vi "main_v1.2.vi"() -> ()   [LabVIEW 2012]
uses:
  SensorSettingCtl.ctl
  SensorTypes.ctl
  states.ctl
  globalVariables.vi
  <vilib>/Analysis/NI_AALPro.lvlib
panel:
  out "Array":dbl[](array[numeric])
  in  "end edge / A":dbl=0.5
  in  "start edge / A":dbl=-0.5
  in  "auto slope detect":bool
  out "mean current difference\nto reference / A":dbl[](array[numeric])
  out "charge difference \nto reference / As":dbl[](array[numeric])
  out "lengths of raw times":i32[](array[numeric])
  out "data analysis running":bool
  out "total charge / As":dbl[](array[numeric]) format="%#.2f"
  out "mean current / A":dbl[](array[numeric]) format="%#_5g"
  out "dt":dbl[][](array[numeric])
  out "end-time / s":dbl[](array[numeric]) format="%.3f"
  out "start-time / s":dbl[](array[numeric]) format="%.3f"
  out "calculated sampling rate / s":dbl[](array[numeric]) format="%^#_5e"
  out "zoomed currents":dbl[][](array[numeric])
  out "zoomed times":dbl[][](array[numeric])
  in  "autostart":bool=TRUE
  out "raw currents":dbl[][](array[numeric])
  in  "start-index":i32[](array[numeric]) min=0 step=1
  in  "end-index":i32[](array[numeric])
  out "raw times":dbl[][](array[numeric])
  in  "exit program":bool
  out "meas. time / s":dbl format="%#.1f"
  in  "max. meas. time / s":dbl=8000.0
  out "measuring":bool
  out "currents raw":cluster{dbl[], dbl[]}[](graph)
  out "currents zoomed":cluster{dbl[], dbl[]}[](graph)
  in  "size of result buffer":i32=400000
  in  "Sensor types":T1[](array[typedef])=[enum."IT 600-S (Analogue)", enum."CAB 300-C SP3 (CAN)", enum."difference"]
  in  "Sensor-enabling":T2[](array[typedef])=[{"VISA resource name"="USB0::0x0957::0x2007::MY49004365::INSTR", "use sensor"=TRUE}, {"VISA resource name"="", "use sensor"=TRUE}]
  in  "stop measurement":bool
  in  "start Button":bool
  out "Error Flag":bool
  # "Measurement of Current Sensors from LEM"
  # "Preparation"
  # "reference"
  # "sensor 1"
  # "sensor 2"
  # "Measurement"
  # "Data analysis"
  # "reference"
  # "sensor 1"
  # "sensor 2"
  # "sensor 3"
  # "sensor 4"
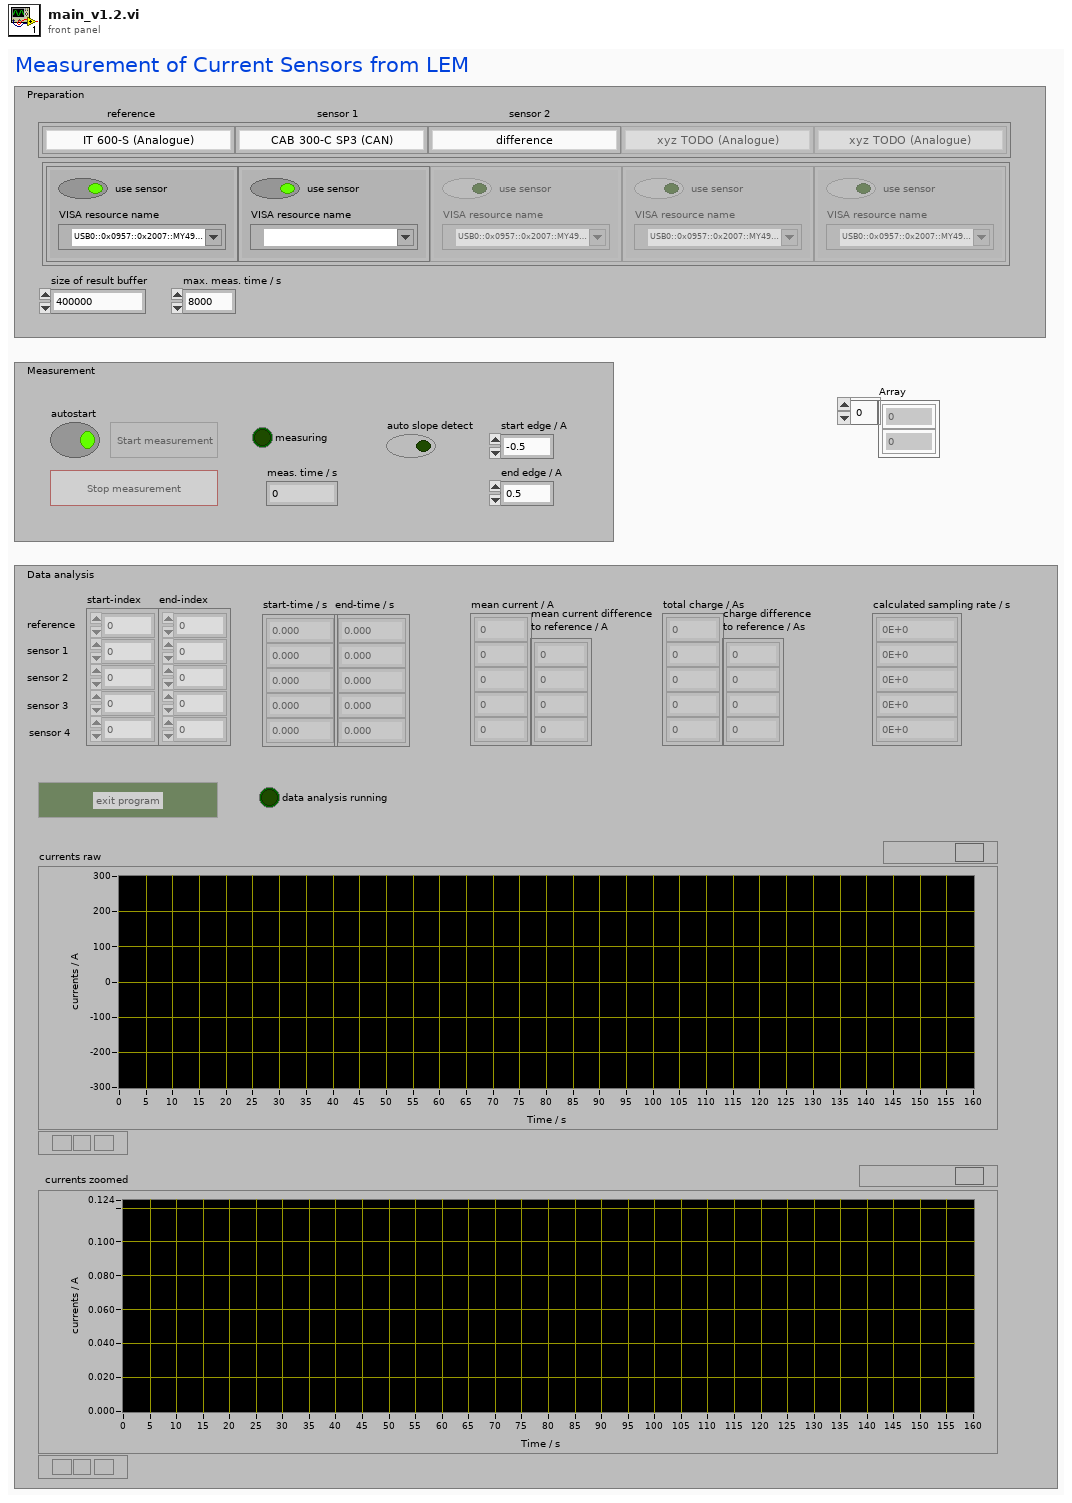
[diagram p1: front panel]
types:
  T1 = typedef "SensorTypes.ctl" = enum16{"IT 600-S (Analogue)", "CAB 300-C SP3 (CAN)", "xyz TODO (PWM)", "xyz TODO (LIN)", "xyz TODO (Analogue)", "difference"}
  T2 = typedef "SensorSettingCtl.ctl" = cluster{"VISA resource name":refnum<visa-resource-name>, "use sensor":bool}
  T3 = typedef "states.ctl" = enum16{"init", "wait for user confirm", "start sensors", "measure", "wait for sensors to finish", "data preparation", "data analysis", "terminate"}
  T4 = enum8{"Enabled", "Disabled", "Disabled and Grayed Out"}
  T5 = typedef "Semaphore RefNum" = refnum<k1>
  T6 = typedef "TimeValue.ctl" = cluster{"Time of measurement":timestamp, "Current value":dbl}
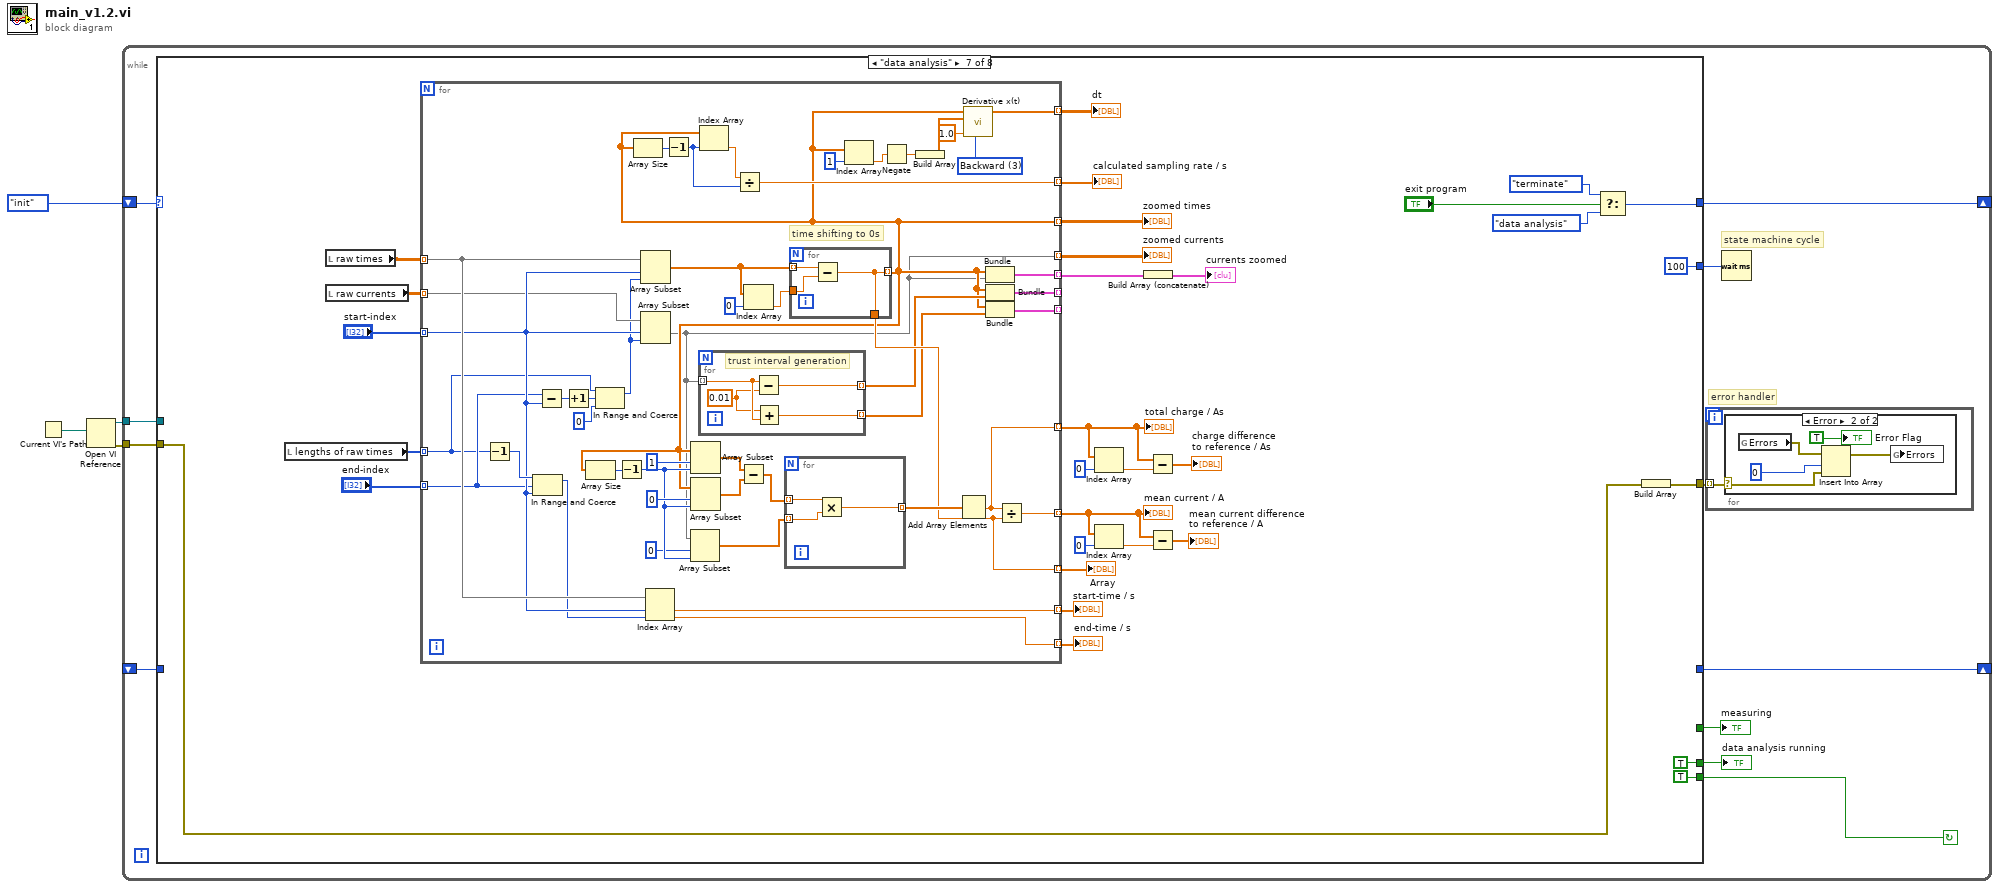
[diagram p0: block diagram]
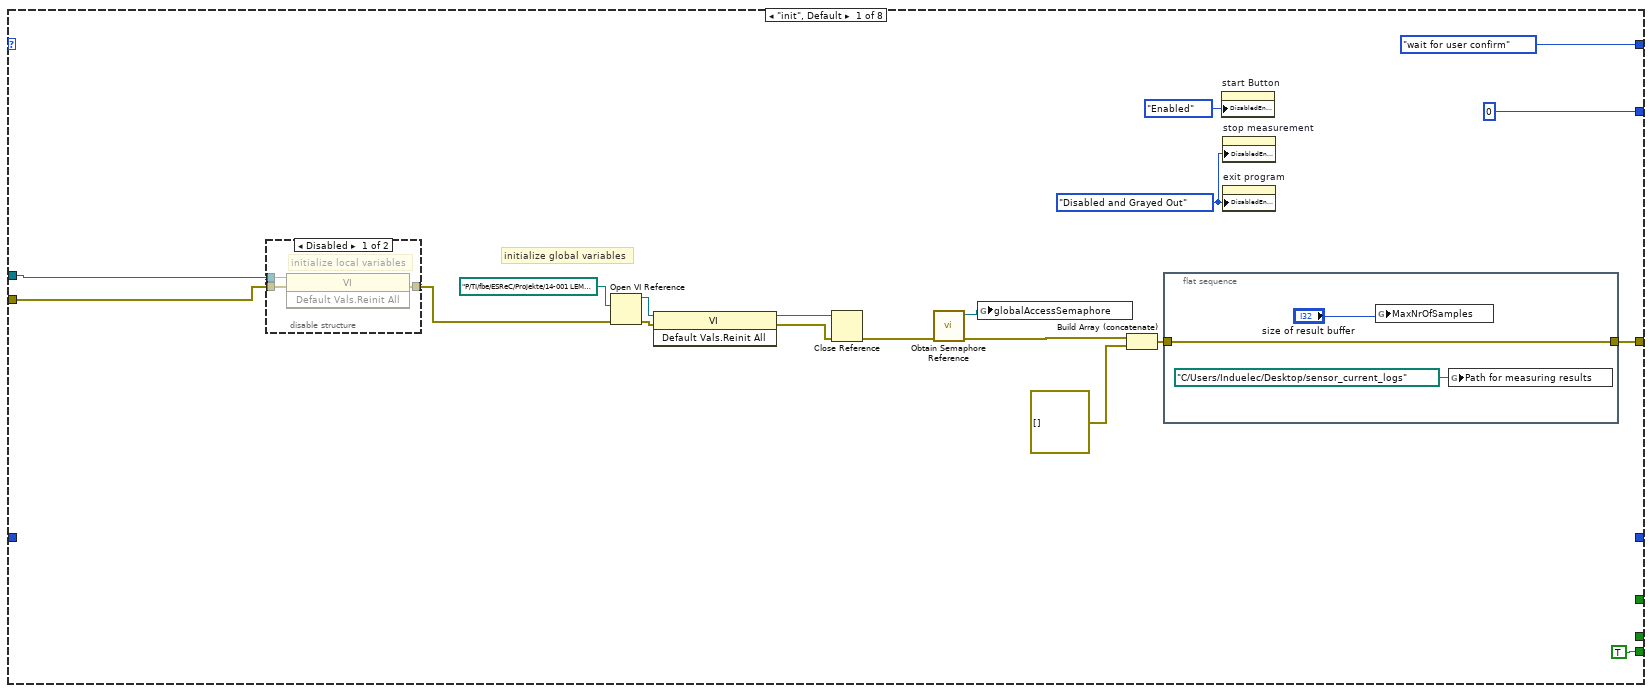
[diagram p3: hidden frame]
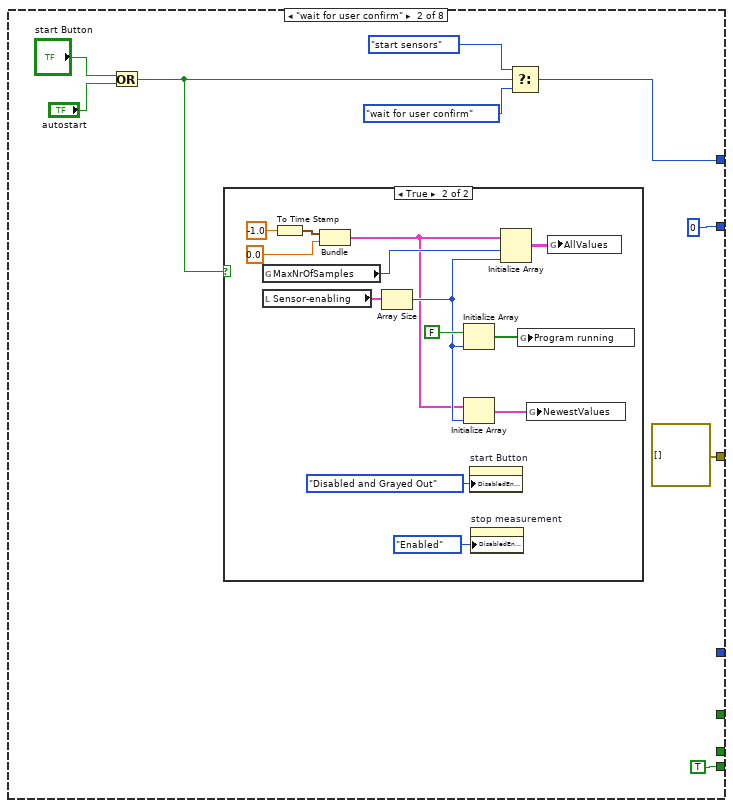
[diagram p5: hidden frame]
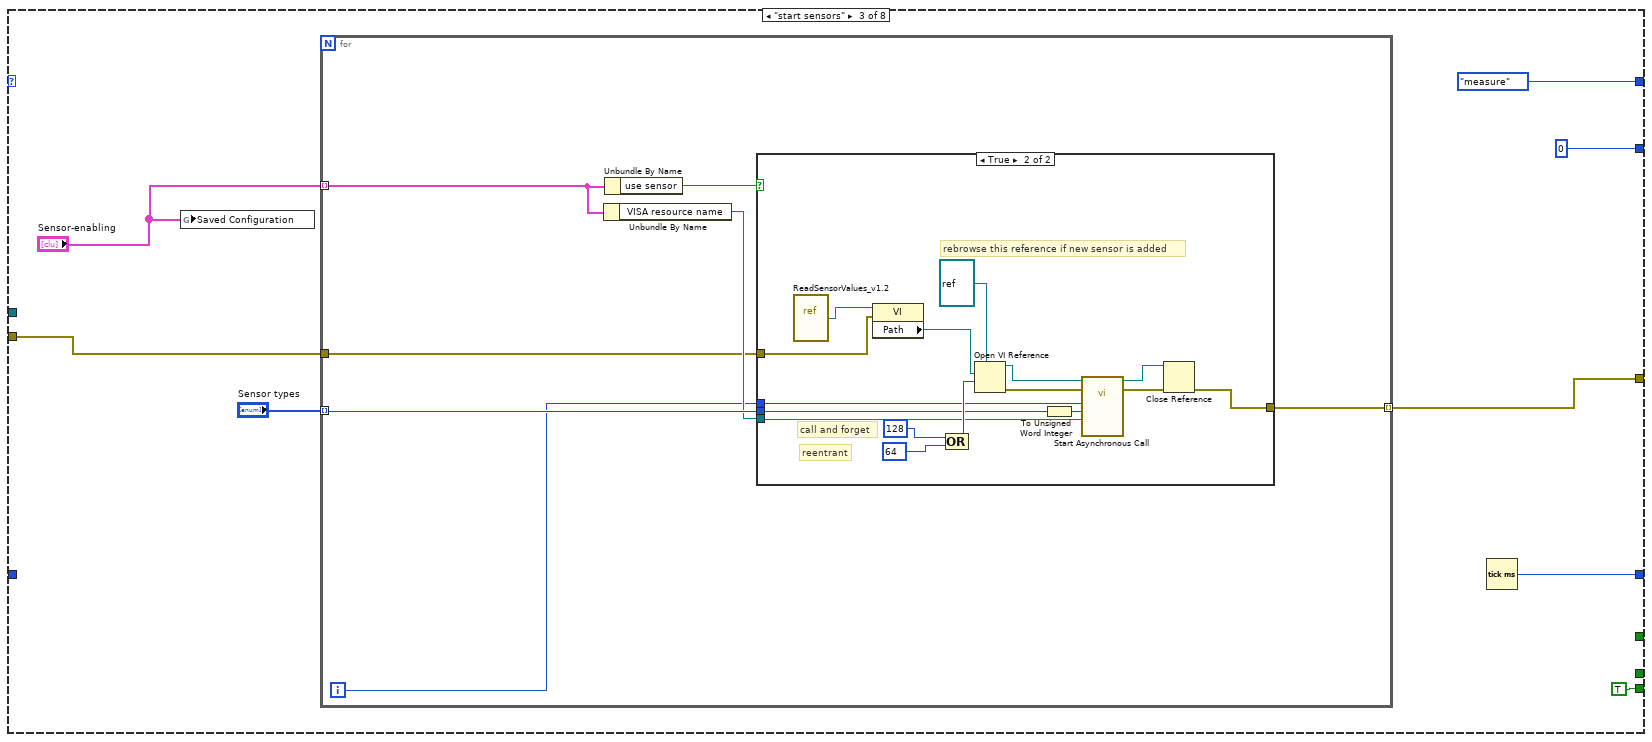
[diagram p7: hidden frame]
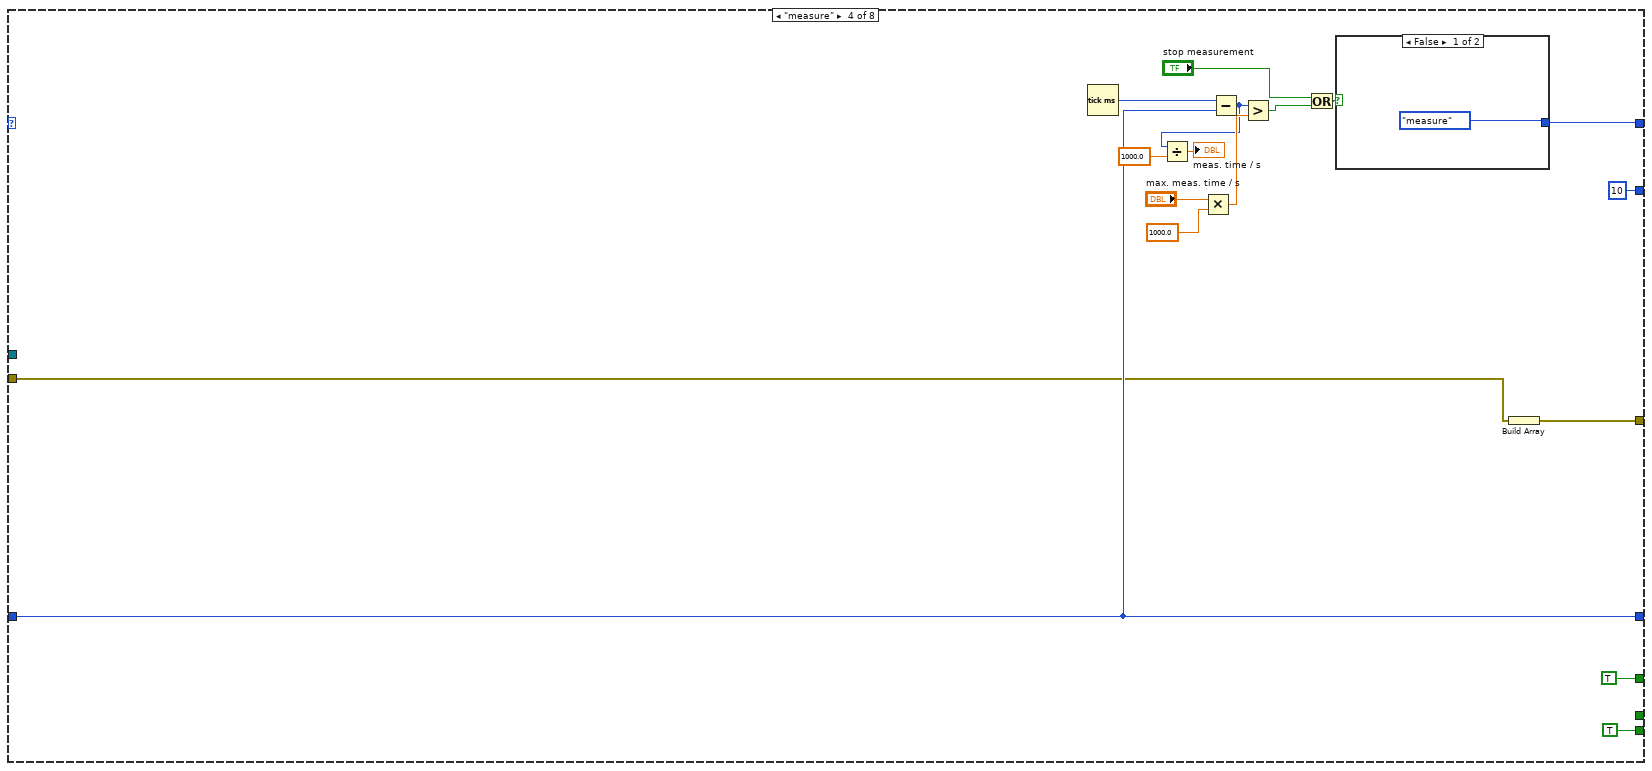
[diagram p9: hidden frame]
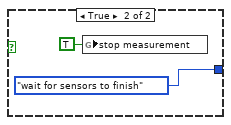
[diagram p10: hidden frame]
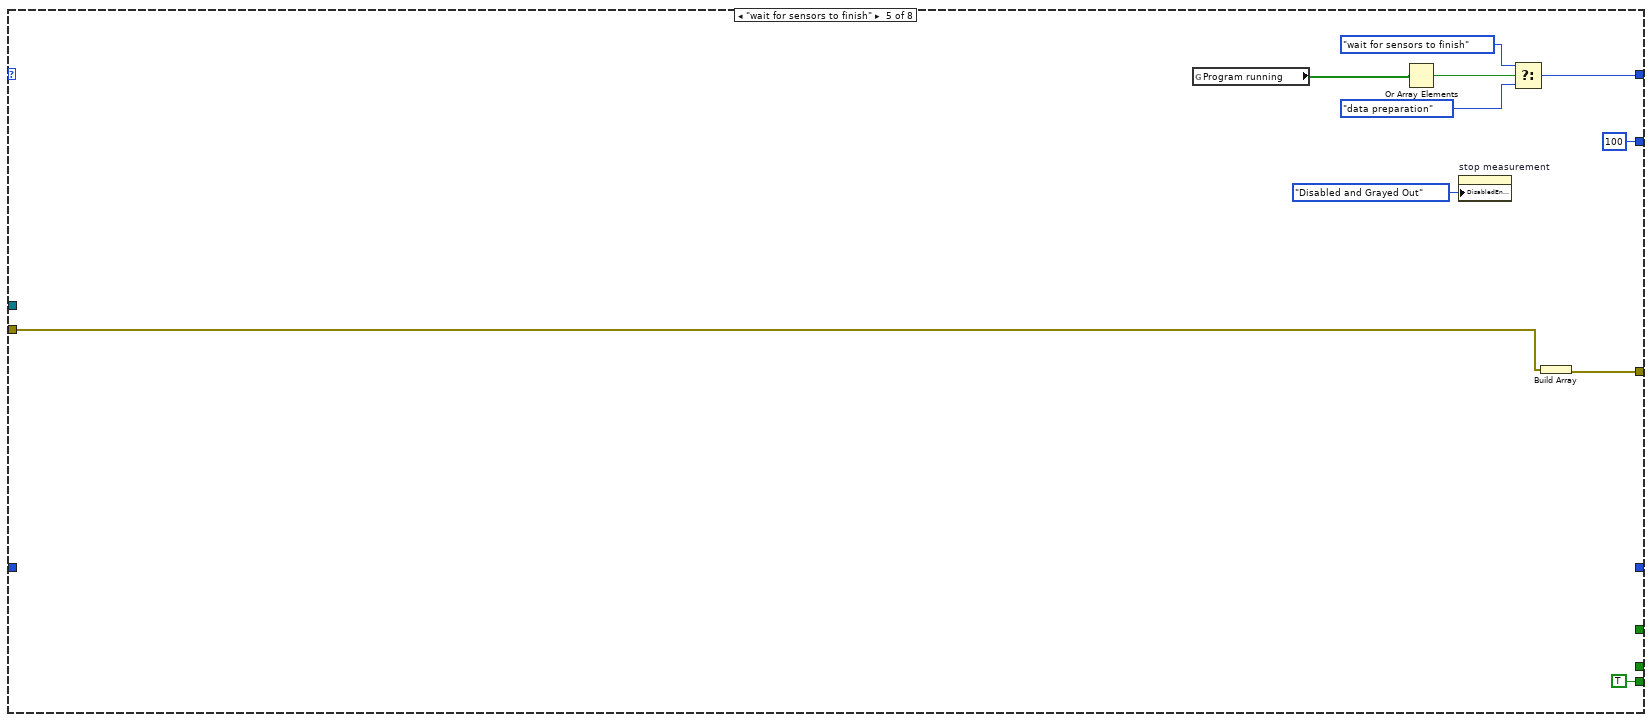
[diagram p11: hidden frame]
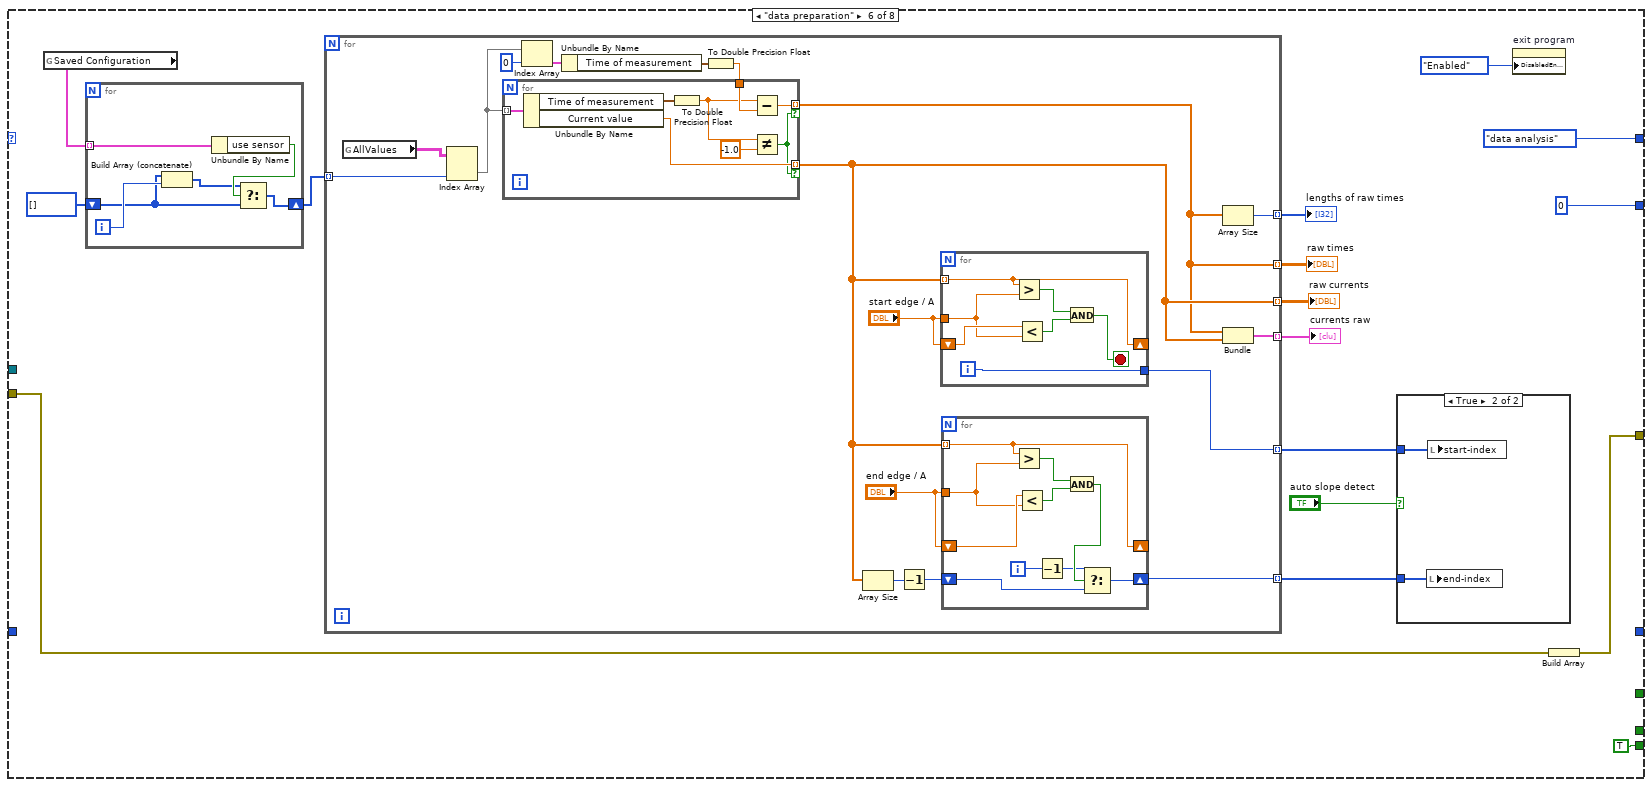
[diagram p12: hidden frame]
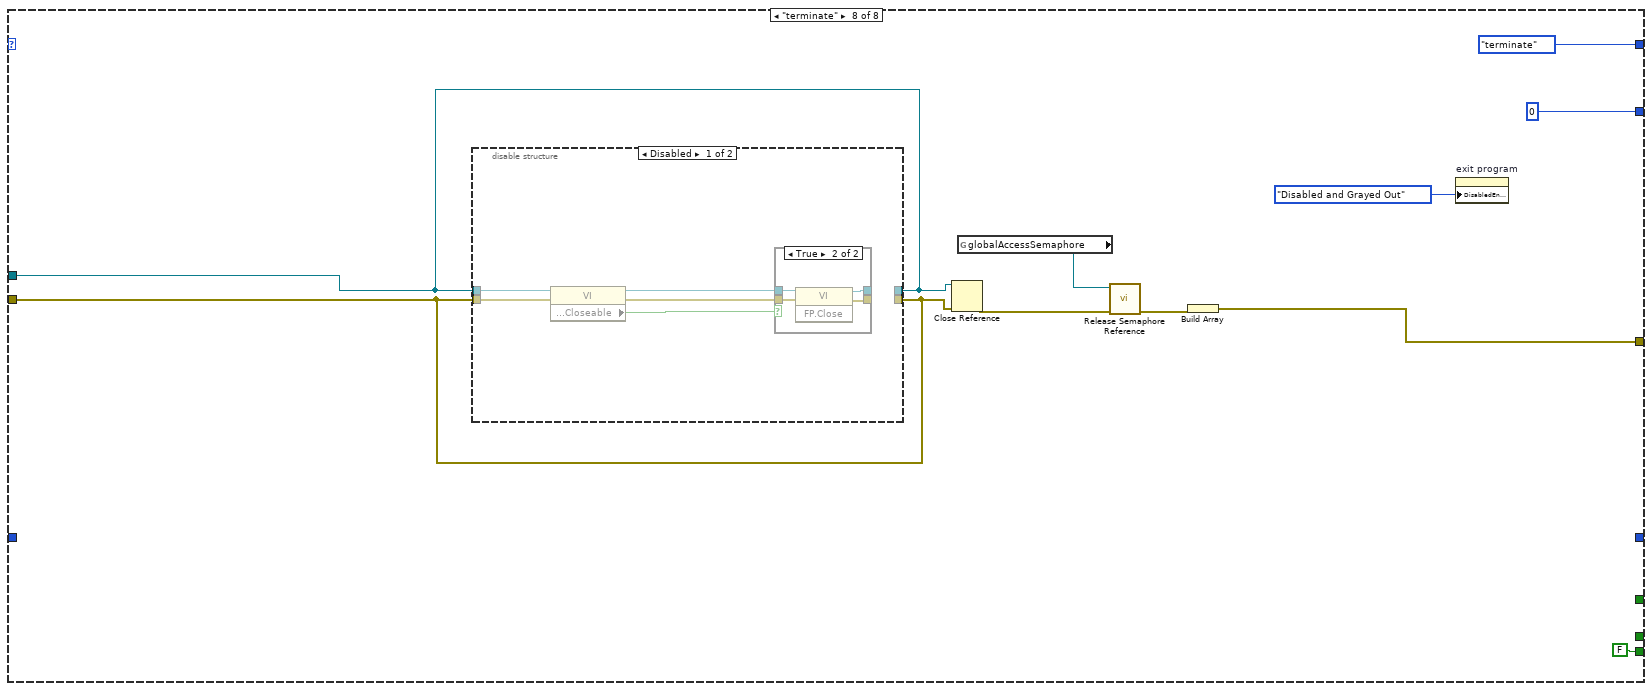
[diagram p14: hidden frame]
diagram:
  n1 = Current VI's Path() -> (path=w4:path)
  n2 = Open VI Reference(vi path=w4) -> (vi reference=w3:refnum<vi>, error out=w2:errorcluster)  [unwired: 2 in, 3 out]
  n3 = while {
    tunnel: w3 -> [w14]
    tunnel: w2 -> [w13]
    shift-right: [w10] -> _
    shift-left: states."init" ("States IEEE-488") -> [w11]
    shift-right: [w8] -> _
    shift-left: _ -> [w7]
    stop <- w9 continue-if-true
    # "error handler"
    # "state machine cycle"
    n4 = case shown="\"data analysis\"" w11 {
      tunnel: [u32 0 ("milliseconds to wait") u32 0 ("milliseconds to wait") u32 0 ("milliseconds to wait") u32 10 ("milliseconds to wait") u32 100 ("milliseconds to wait") u32 0 ("milliseconds to wait") u32 100 ("milliseconds to wait") u32 0 ("milliseconds to wait")] -> w15
      tunnel: w14 -> [w38 _ _ _ _ _ _ w290]
      tunnel: w13 -> [w39 _ w70 w101 w123 w144 w220 w289]
      tunnel: [w24 errorcluster[] [] w74 w102 w124 w145 w221 w293] -> w12
      tunnel: [states."wait for user confirm" ("States IEEE-488") w53 states."measure" ("States IEEE-488") w117 w126 states."data analysis" ("f") w199 states."terminate" ("f")] -> w10
      tunnel: [TRUE TRUE TRUE TRUE TRUE TRUE TRUE FALSE] -> w9
      tunnel: [_ _ w69 w112 _ _ _ _] -> w8
      tunnel: w7 -> [_ _ _ w112 _ _ _ _]
      tunnel: [_ _ _ TRUE ("measuring") _ _ _ _] -> w6
      tunnel: [_ _ _ _ _ _ TRUE ("measuring") _] -> w5
      frame "init", Default {
        w22 = T4."Disabled and Grayed Out" ("Disabled")
        # "initialize global variables"
        n5 = disable-structure shown="Disabled" {
          disable-tunnel: w39 -> [w46 _]
          disable-tunnel: w38 -> [w45 _]
          disable-tunnel: [w44 _] -> w32
          frame Disabled {
            # "initialize local variables"
            n6 = invoke class="VI" method="Default Vals.Reinit All"(reference=w45, error in=w46) -> (error out=w44:errorcluster)  [unwired: 1 in, 2 out]
          }
          frame Enabled {
          }
        }
        n7 = Open VI Reference(vi path=path "P:/TI/fbe/ESReC/Projekte/14-001 LEM Current Sensor Measurements/Software/LabVIEW/Current sensor tests/globalVariables.vi", error in (no error)=w32) -> (vi reference=w33:refnum<vi>, error out=w31:errorcluster)  [unwired: 4 in]
        n8 = invoke class="VI" method="Default Vals.Reinit All"(reference=w33, error in=w31) -> (reference out=w30:refnum<vi>, error out=w29:errorcluster)  [unwired: 1 in, 1 out]
        n9 = Close Reference(reference=w30, error in (no error)=w29) -> (error out=w27:errorcluster)
        n10 = call <vilib>:"Obtain Semaphore Reference.vi"("error in (no error)"=w27) -> ("error out"=w26:errorcluster, "semaphore"=w28:T5)  [unwired: 4 in, 1 out]
        n11 = global write "globalVariables.vi" "globalAccessSemaphore"(w28) -> ()
        n12 = Build Array (concatenate)(w26, errorcluster[] [] ("array")) -> (w25:errorcluster[])
        n13 = flat-sequence {
          tunnel: w25 -> [w42]
          tunnel: [w42] -> w24
          frame #0 {
            n14 = global write "globalVariables.vi" "MaxNrOfSamples"("size of result buffer") -> ()
            n15 = global write "globalVariables.vi" "Path for measuring results"(path "C:/Users/Induelec/Desktop/sensor_current_logs" ("Path for measuring results")) -> ()
          }
        }
        n16 = property on="start Button" class="Bool (strict)"("DisabledEnum"=T4."Enabled" ("Disabled")) -> ()  [unwired: 2 in, 2 out]
        n17 = property on="stop measurement" class="Bool"("DisabledEnum"=w22) -> ()  [unwired: 2 in, 2 out]
        n18 = property on="exit program" class="Bool"("DisabledEnum"=w22) -> ()  [unwired: 2 in, 2 out]
      }
      frame "wait for user confirm" {
        n19 = Or(x="start Button", y="autostart") -> (x .or. y?=w47:bool)
        n20 = case shown="True" w47 {
          frame False {
          }
          frame True {
            n21 = global read "globalVariables.vi" "MaxNrOfSamples"() -> (w64:i32)
            n22 = local read "Sensor-enabling"() -> (w63:T2[])
            n23 = To Time Stamp(1:-1.0 ("number")) -> (0:w66:timestamp)
            n24 = Bundle(w66, 0.0) -> (w56:cluster{timestamp, dbl})  [unwired: 1 in]
            n25 = Array Size(array=w63) -> (size(s)=w58:i32)
            n26 = Initialize Array(FALSE ("Boolean"), w58) -> (w62:bool[])
            n27 = Initialize Array(w56, w58) -> (w57:cluster{timestamp, dbl}[])
            n28 = property on="start Button" class="Bool (strict)"("DisabledEnum"=T4."Disabled and Grayed Out" ("Disabled")) -> ()  [unwired: 2 in, 2 out]
            n29 = property on="stop measurement" class="Bool"("DisabledEnum"=T4."Enabled" ("Disabled")) -> ()  [unwired: 2 in, 2 out]
            n30 = Initialize Array(w56, w64, w58) -> (w68:cluster{timestamp, dbl}[][])
            n31 = global write "globalVariables.vi" "Program running"(w62) -> ()
            n32 = global write "globalVariables.vi" "NewestValues"(w57) -> ()
            n33 = global write "globalVariables.vi" "AllValues"(w68) -> ()
          }
        }
        n34 = Select(t=states."start sensors" ("States IEEE-488"), s=w47, f=states."wait for user confirm" ("States IEEE-488")) -> (s? t:f=w53:T3)
      }
      frame "start sensors" {
        n35 = global write "globalVariables.vi" "Saved Configuration"("Sensor-enabling") -> ()
        n36 = for {
          tunnel: "Sensor-enabling" -> [w82] mode=indexing
          tunnel: [w81] -> w74 mode=indexing
          tunnel: "Sensor types" -> [w80] mode=indexing
          tunnel: w70 -> [w78]
          i -> [w77]
          n37 = Unbundle By Name(w82) -> ("VISA resource name"=w79:refnum<visa-resource-name>)
          n38 = Unbundle By Name(w82) -> ("use sensor"=w83:bool)
          n39 = case shown="True" w83 {
            tunnel: [w84 w98] -> w81
            tunnel: w80 -> [_ w85]
            tunnel: w79 -> [_ w91]
            tunnel: w78 -> [w84 w92]
            tunnel: w77 -> [_ w87]
            frame False {
            }
            frame True {
              # "rebrowse this reference if new sensor is added"
              # "reentrant"
              # "call and forget"
              n40 = vi-ref "ReadSensorValues_v1.2.vi"() -> (w89:refnum<vi>)
              n41 = property class="VI"(reference=w89, error in=w92) -> ("Path"=w100:path)  [unwired: 2 out]
              n42 = Compound Arithmetic op=OR(128 ("options"), 64 ("value")) -> (w97:i32)
              n43 = Open VI Reference(type specifier VI Refnum (for type only)=refnum<vi> refnum, vi path=w100, options=w97) -> (vi reference=w88:refnum<vi>, error out=w95:errorcluster)  [unwired: 3 in]
              n44 = To Unsigned Word Integer(number=w85) -> (unsigned 16bit integer=w86:u16)
              n45 = call-by-ref "Start Asynchronous Call"(reference=w88, error in=w95, "VISA resource name"=w91, "sensor type nr"=w86, "Sensor Nr"=w87) -> (reference out=w94:refnum<vi>, error out=w93:errorcluster)  [unwired: 1 in]
              n46 = Close Reference(reference=w94, error in (no error)=w93) -> (error out=w98:errorcluster)
            }
          }
        }
        n47 = Tick Count (ms)() -> (millisecond timer value=w69:u32)
      }
      frame "measure" {
        n48 = Tick Count (ms)() -> (millisecond timer value=w107:u32)
        n49 = Multiply(x="max. meas. time / s", y=1000.0) -> (x*y=w110:dbl)
        n50 = Subtract(x=w107, y=w112) -> (x-y=w105:u32)
        n51 = Divide(x=w105, y=1000.0) -> (x/y=→"meas. time / s":dbl)
        n52 = Greater?(x=w105, y=w110) -> (0:w113:bool)
        n53 = Or(x="stop measurement", y=w113) -> (x .or. y?=w115:bool)
        n54 = case shown="False" w115 {
          tunnel: [states."measure" ("f") states."wait for sensors to finish" ("States IEEE-488")] -> w117
          frame False {
          }
          frame True {
            n55 = global write "globalVariables.vi" "stop measurement"(TRUE ("stop measurement")) -> ()
          }
        }
        n56 = Build Array(w101) -> (w102:errorcluster[])
      }
      frame "wait for sensors to finish" {
        n57 = global read "globalVariables.vi" "Program running"() -> (w130:bool[])
        n58 = Or Array Elements(Boolean array=w130) -> (logical OR=w128:bool)
        n59 = property on="stop measurement" class="Bool"("DisabledEnum"=T4."Disabled and Grayed Out" ("Disabled")) -> ()  [unwired: 2 in, 2 out]
        n60 = Select(t=states."wait for sensors to finish" ("States IEEE-488"), s=w128, f=states."data preparation" ("States IEEE-488")) -> (s? t:f=w126:T3)
        n61 = Build Array(w123) -> (w124:errorcluster[])
      }
      frame "data preparation" {
        n62 = global read "globalVariables.vi" "Saved Configuration"() -> (w136:T2[])
        n63 = for {
          tunnel: w136 -> [w154] mode=indexing
          shift-right: [w152] -> w135
          shift-left: i32[] [] -> [w149]
          i -> [w150]
          n64 = Build Array (concatenate)(w149, w150) -> (w151:i32[])
          n65 = Unbundle By Name(w154) -> ("use sensor"=w153:bool)
          n66 = Select(t=w151, s=w153, f=w149) -> (s? t:f=w152:i32[])
        }
        n67 = for {
          tunnel: w135 -> [w166] mode=indexing
          tunnel: [w156] -> w138 mode=indexing
          tunnel: [w158] -> w141 mode=indexing
          tunnel: [w160] -> w142 mode=indexing
          tunnel: [w159] -> w132 mode=indexing
          tunnel: [w157] -> w140 mode=indexing
          tunnel: [w155] -> w137 mode=indexing
          n68 = global read "globalVariables.vi" "AllValues"() -> (w171:T6[][])
          n69 = Index Array(array=w171, index (col)=w166) -> (element=w165:T6[])  [unwired: 1 in]
          n70 = Index Array(array=w165, index=0) -> (element=w169:T6)
          n71 = Unbundle By Name(w169) -> ("Time of measurement"=w168:timestamp)
          n72 = To Double Precision Float(number=w168) -> (double precision float=w167:dbl)
          n73 = for {
            tunnel: w165 -> [w196] mode=indexing
            tunnel: [w189] -> w156 mode=indexing if=w190
            tunnel: [w194] -> w158 mode=indexing if=w190
            tunnel: w167 -> [w193]
            n74 = Unbundle By Name(w196) -> ("Time of measurement"=w195:timestamp, "Current value"=w194:dbl)
            n75 = To Double Precision Float(number=w195) -> (double precision float=w191:dbl)
            n76 = Subtract(x=w191, y=w193) -> (x-y=w189:dbl)
            n77 = Not Equal?(x=w191, y=-1.0) -> (x != y?=w190:bool)
          }
          n78 = Array Size(array=w158) -> (size(s)=w164:i32)
          n79 = Decrement(x=w164) -> (x-1=w163:i32)
          n80 = for {
            tunnel: w158 -> [w184] mode=indexing
            tunnel: [w188] -> w159
            shift-right: [w184] -> _
            shift-left: "start edge / A" -> [w183]
            tunnel: "start edge / A" -> [w182]
            i -> [w188]
            stop <- w186 stop-if-true
            n81 = Greater?(x=w184, y=w182) -> (0:w185:bool)
            n82 = Less?(x=w183, y=w182) -> (x < y?=w187:bool)
            n83 = And(x=w185, y=w187) -> (x .and. y?=w186:bool)
          }
          n84 = for {
            tunnel: w158 -> [w176] mode=indexing
            shift-right: [w181] -> w160
            shift-left: w163 -> [w180]
            shift-right: [w176] -> _
            shift-left: "end edge / A" -> [w175]
            tunnel: "end edge / A" -> [w174]
            i -> [w173]
            n85 = Greater?(x=w176, y=w174) -> (0:w179:bool)
            n86 = Less?(x=w175, y=w174) -> (x < y?=w178:bool)
            n87 = Decrement(x=w173) -> (x-1=w172:i32)
            n88 = And(x=w179, y=w178) -> (x .and. y?=w177:bool)
            n89 = Select(t=w172, s=w177, f=w180) -> (s? t:f=w181:i32)
          }
          n90 = Array Size(array=w156) -> (size(s)=w155:i32)
          n91 = Bundle(w156, w158) -> (w157:cluster{dbl[], dbl[]})  [unwired: 1 in]
        }
        "raw times" <- w138
        "currents raw" <- w140
        "raw currents" <- w141
        "lengths of raw times" <- w137
        n92 = case shown="True" "auto slope detect" {
          tunnel: w142 -> [_ w148]
          tunnel: w132 -> [_ w147]
          frame False {
          }
          frame True {
            n93 = local write "end-index"(w148) -> ()
            n94 = local write "start-index"(w147) -> ()
          }
        }
        n95 = property on="exit program" class="Bool"("DisabledEnum"=T4."Enabled" ("Disabled")) -> ()  [unwired: 2 in, 2 out]
        n96 = Build Array(w144) -> (w145:errorcluster[])
      }
      frame "data analysis" {
        n97 = local read "lengths of raw times"() -> (w210:i32[])
        n98 = local read "raw times"() -> (w225:dbl[][])
        n99 = local read "raw currents"() -> (w224:dbl[][])
        n100 = for {
          tunnel: "start-index" -> [w240] mode=indexing
          tunnel: "end-index" -> [w237] mode=indexing
          tunnel: w225 -> [w246] mode=indexing
          tunnel: w224 -> [w239] mode=indexing
          tunnel: [w272] -> w223 mode=indexing
          tunnel: [w271] -> _ mode=indexing
          tunnel: [w270] -> _ mode=indexing
          tunnel: [w229] -> w214 mode=indexing
          tunnel: [w228] -> w218 mode=indexing
          tunnel: [w248] -> w216 mode=indexing
          tunnel: [w247] -> w215 mode=indexing
          tunnel: [w261] -> w213 mode=indexing
          tunnel: [w249] -> w203 mode=indexing
          tunnel: [w245] -> w207 mode=indexing
          tunnel: [w241] -> w212 mode=indexing
          tunnel: w210 -> [w234] mode=indexing
          tunnel: [w232] -> w197 mode=indexing
          w266 = u16 3 items=["2nd Order Central", "4th Order Central", "Forward", "Backward"] ("method")
          # "time shifting to 0s"
          n101 = Decrement(x=w234) -> (x-1=w274:i32)
          n102 = In Range and Coerce(upper limit=w274, x=w237, lower limit=w240) -> (coerced(x)=w238:i32)  [unwired: 1 out]
          n103 = Subtract(x=w237, y=w240) -> (x-y=w269:i32)
          n104 = Increment(x=w269) -> (x+1=w235:i32)
          n105 = In Range and Coerce(upper limit=w234, x=w235, lower limit=0) -> (coerced(x)=w236:i32)  [unwired: 1 out]
          n106 = Array Subset(array=w246, index=w240, length=w236) -> (w258:dbl[])
          n107 = Array Subset(array=w239, index=w240, length=w236) -> (w228:dbl[])
          n108 = Index Array(array=w246, index #1=w240, index #2=w238) -> (element #1=w248:dbl, element #2=w247:dbl)
          n109 = for {
            tunnel: w228 -> [w284] mode=indexing
            tunnel: [w282] -> w230 mode=indexing
            tunnel: [w281] -> w231 mode=indexing
            w283 = 0.01
            # "trust interval generation"
            n110 = Subtract(x=w284, y=w283) -> (x-y=w282:dbl)
            n111 = Add(x=w283, y=w284) -> (x+y=w281:dbl)
          }
          n112 = Index Array(array=w258, index=0) -> (element=w268:dbl)
          n113 = for {
            tunnel: w268 -> [w279]
            tunnel: w258 -> [w280] mode=indexing
            tunnel: [w278] -> w229 mode=indexing
            tunnel: [w278] -> w232
            n114 = Subtract(x=w280, y=w279) -> (x-y=w278:dbl)
          }
          n115 = Array Size(array=w229) -> (size(s)=w259:i32)
          n116 = Decrement(x=w259) -> (x-1=w254:i32)
          n117 = Array Size(array=w229) -> (size(s)=w243:i32)
          n118 = Decrement(x=w243) -> (x-1=w242:i32)
          n119 = Array Subset(array=w228, index=0, length=w254) -> (w251:dbl[])
          n120 = Array Subset(array=w229, index=1, length=w254) -> (w256:dbl[])
          n121 = Array Subset(array=w229, index=0, length=w254) -> (w255:dbl[])
          n122 = Index Array(array=w229, index=w242) -> (element=w244:dbl)
          n123 = Divide(x=w244, y=w242) -> (x/y=w241:dbl)
          n124 = Subtract(x=w256, y=w255) -> (x-y=w252:dbl[])
          n125 = for {
            tunnel: w252 -> [w277] mode=indexing
            tunnel: w251 -> [w276] mode=indexing
            tunnel: [w275] -> w250 mode=indexing
            n126 = Multiply(x=w277, y=w276) -> (x*y=w275:dbl)
          }
          n127 = Index Array(array=w229, index=1) -> (element=w264:dbl)
          n128 = Negate(x=w264) -> (-x=w263:dbl)
          n129 = Build Array(w263) -> (w262:dbl[])
          n130 = Add Array Elements(numeric array=w250) -> (sum=w245:dbl)
          n131 = call <vilib>:"Derivative x(t).vi"("method"=w266, "dt"=1.0, "Initial Condition"=w262, "X"=w229) -> ("dX/dt"=w261:dbl[])  [unwired: 6 in, 1 out]
          n132 = Bundle(w229, w228) -> (w272:cluster{dbl[], dbl[]})  [unwired: 1 in]
          n133 = Bundle(w229, w230) -> (w271:cluster{dbl[], dbl[]})  [unwired: 1 in]
          n134 = Bundle(w229, w231) -> (w270:cluster{dbl[], dbl[]})  [unwired: 1 in]
          n135 = Divide(x=w245, y=w232) -> (x/y=w249:dbl)
        }
        "zoomed times" <- w214
        "zoomed currents" <- w218
        "start-time / s" <- w216
        "end-time / s" <- w215
        "dt" <- w213
        "mean current / A" <- w203
        "total charge / As" <- w207
        "calculated sampling rate / s" <- w212
        "Array" <- w197
        n136 = Index Array(array=w207, index=0) -> (element=w206:dbl)
        n137 = Index Array(array=w203, index=0) -> (element=w205:dbl)
        n138 = Build Array (concatenate)(w223) -> (→"currents zoomed":cluster{dbl[], dbl[]}[])
        n139 = Subtract(x=w207, y=w206) -> (x-y=→"charge difference \nto reference / As":dbl[])
        n140 = Subtract(x=w203, y=w205) -> (x-y=→"mean current difference\nto reference / A":dbl[])
        n141 = Select(t=states."terminate" ("f"), s="exit program", f=states."data analysis") -> (s? t:f=w199:T3)
        n142 = Build Array(w220) -> (w221:errorcluster[])
      }
      frame "terminate" {
        n143 = disable-structure shown="Disabled" {
          disable-tunnel: w289 -> [w296 _]
          disable-tunnel: w290 -> [w295 _]
          disable-tunnel: w290 -> [_ _]
          disable-tunnel: w289 -> [_ _]
          frame Disabled {
            n144 = property class="VI"(reference=w295, error in=w296) -> (reference out=w298:refnum<vi>, error out=w297:errorcluster, "Front Panel.Closeable"=w299:bool)
            n145 = case shown="True" w299 {
              tunnel: w298 -> [w301 w305]
              tunnel: [w301 w304] -> _
              tunnel: w297 -> [w300 w303]
              tunnel: [w300 w302] -> _
              frame False {
              }
              frame True {
                n146 = invoke class="VI" method="FP.Close"(reference=w305, error in=w303) -> (reference out=w304:refnum<vi>, error out=w302:errorcluster)  [unwired: 1 in, 1 out]
              }
            }
          }
          frame Enabled {
          }
        }
        n147 = Close Reference(reference=w290, error in (no error)=w289) -> (error out=w286:errorcluster)
        n148 = global read "globalVariables.vi" "globalAccessSemaphore"() -> (w288:T5)
        n149 = call <vilib>:"Release Semaphore Reference.vi"("error in (no error)"=w286, "semaphore"=w288) -> ("error out"=w287:errorcluster)  [unwired: 8 in, 1 out]
        n150 = Build Array(w287) -> (w293:errorcluster[])
        n151 = property on="exit program" class="Bool"("DisabledEnum"=T4."Disabled and Grayed Out" ("Disabled")) -> ()  [unwired: 2 in, 2 out]
      }
    }
    "measuring" <- w6
    "data analysis running" <- w5
    n152 = for {
      tunnel: w12 -> [w16] mode=indexing
      n153 = case shown="Error" w16 {
        selector: w16 -> [_ w20]
        frame No Error {
        }
        frame Error {
          n154 = global read "globalVariables.vi" "Errors"() -> (w18:errorcluster[])
          n155 = Insert Into Array(array=w18, index=0, new element=w20) -> (w17:errorcluster[])
          n156 = global write "globalVariables.vi" "Errors"(w17) -> ()
          "Error Flag" <- TRUE ("Error Flag")
        }
      }
    }
    n157 = Wait (ms)(milliseconds to wait=w15) -> ()  [unwired: 1 out]
  }
